vi "Login Credentials Dialog.vi"(8 "Error In":errorcluster, 10 "Password In":string, 11 "Username In":string) -> (0 "Error Out":errorcluster, 2 "Password Out":string, 3 "Username Out":string)   [LabVIEW 2017, in "Tests.lvlib"]
uses:
  Tests.lvlib
panel:
  in  "Cancel":bool
  in  "OK":bool
  in  "Password":string
  in  "Username":string
  # "SSH TEST SERVER LOGIN"
  # "PASSWORD:"
  # "USERNAME:"
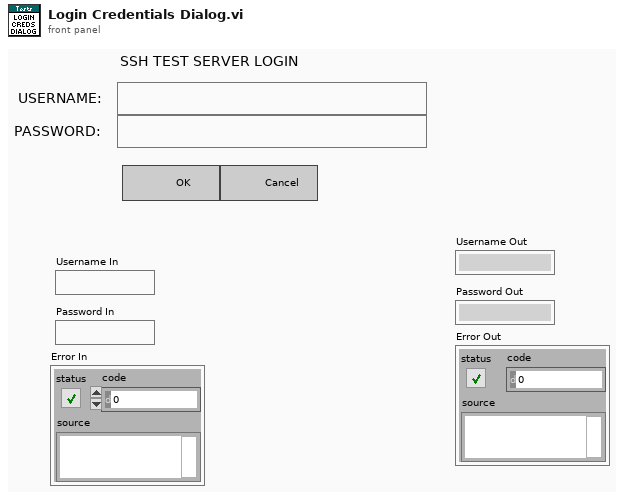
[diagram p1: front panel]
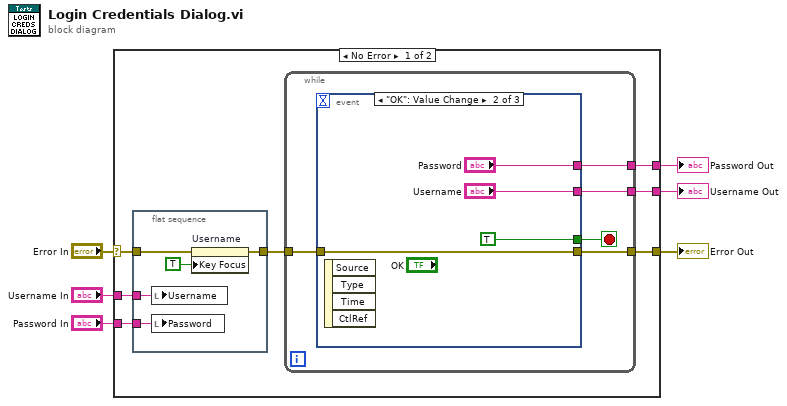
[diagram p0: block diagram]
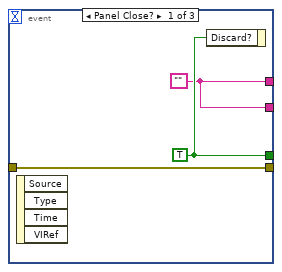
[diagram p2: hidden frame]
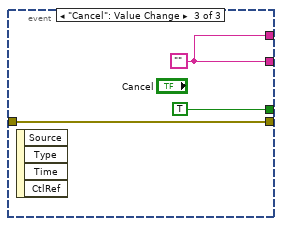
[diagram p3: hidden frame]
diagram:
  n1 = case shown="No Error" "Error In" {
    selector: "Error In" -> [w10 w34]
    tunnel: [w13 w34] -> w5
    tunnel: [w7 _] -> w4
    tunnel: [w8 _] -> w3
    tunnel: "Password In" -> [w11 _]
    tunnel: "Username In" -> [w12 _]
    frame No Error {
      n2 = flat-sequence {
        tunnel: w12 -> [w18]
        tunnel: w11 -> [w17]
        tunnel: w10 -> [w16]
        tunnel: [w15] -> w9
        frame #0 {
          n3 = local write "Username"(w18) -> ()
          n4 = local write "Password"(w17) -> ()
          n5 = property on="Username" class="Str"(error in=w16, "Key Focus"=TRUE) -> (error out=w15:errorcluster)  [unwired: 1 in, 1 out]
        }
      }
      n6 = while {
        tunnel: w9 -> [w22]
        tunnel: [w21] -> w13
        tunnel: [w20] -> w8
        tunnel: [w19] -> w7
        stop <- w23 stop-if-true
        n7 = event shown="[1] \"OK\": Value Change" {
          selector: _ -> [_ _ _]
          dyn-events: _ -> [_ _ _]
          timeout: _ -> [_ _ _]
          tunnel: [w26 TRUE TRUE] -> w23
          tunnel: w22 -> [w25 w30 w33]
          tunnel: [w25 w30 w33] -> w21
          tunnel: [w24 "Password" w31] -> w20
          tunnel: [w24 "Username" w31] -> w19
          event Panel Close? {
            w24 = ""
            w26 = TRUE
            n8 = event-data() -> ()  [unwired: 1 in, 4 out]
            n9 = event-data("Discard?"=w26) -> ()  [unwired: 1 in, 1 out]
          }
          event "OK": Value Change {
            n10 = event-data() -> ()  [unwired: 1 in, 4 out]
          }
          event "Cancel": Value Change {
            w31 = ""
            n11 = event-data() -> ()  [unwired: 1 in, 4 out]
          }
        }
      }
    }
    frame Error {
    }
  }
  "Error Out" <- w5
  "Username Out" <- w4
  "Password Out" <- w3
